vi "List Attribute Names.vi"(7 "Tree ID":string, 8 "Error In":errorcluster, 11 "Tree Manager":refnum<data-value>) -> (0 "Error Out":errorcluster, 1 "Attribute Names":string[](array[string]), 3 "Tree Manager":refnum<data-value>)   [LabVIEW 2017, in "Tree API.lvlib" / "Tree.lvclass"]
doc: "List the attributes names for the specified Tree.\n\nThe list order is preserved as defined."
uses:
  Tree.lvclass
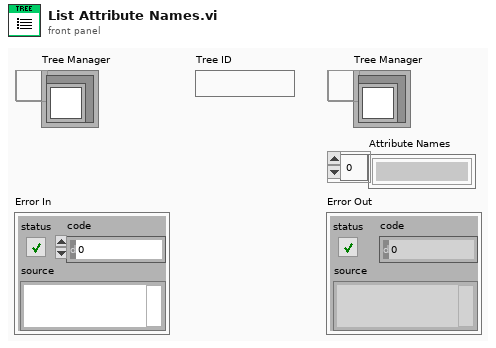
[diagram p1: front panel]
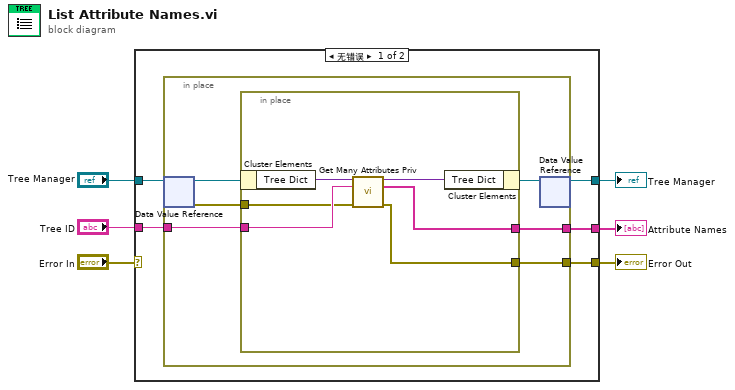
[diagram p0: block diagram]
diagram:
  n1 = case shown="无错误" "Error In" {
    selector: "Error In" -> [_ w24]
    tunnel: "Tree Manager" -> [w11 w25]
    tunnel: [w10 w25] -> w5
    tunnel: [w9 w24] -> w3
    tunnel: "Tree ID" -> [w8 _]
    tunnel: [w7 _] -> w1
    frame No Error {
      n2 = in-place {
        in-place-border: [w16] -> w9
        in-place-border: w8 -> [w13]
        in-place-border: [w12] -> w7
        n3 = in-place-dvr #1(w11) -> (w17:refnum<class "Tree.lvclass">, w14:errorcluster)
        n4 = in-place {
          in-place-border: [w19] -> w16
          in-place-border: w14 -> [w21]
          in-place-border: w13 -> [w22]
          in-place-border: [w18] -> w12
          n5 = in-place-cluster #2(w17) -> ("Tree Dict"=w23:variant)
          n6 = call "Get Many Attributes Priv.vi"("Tree Dictionary In"=w23, "Unique ID"=w22, "error in"=w21) -> ("Tree Dictionary Out"=w20:variant, "Attribute Names"=w18:string[], "error out"=w19:errorcluster)  [unwired: 7 in, 3 out]
          n7 = in-place-cluster #2("Tree Dict"=w20) -> (w15:refnum<class "Tree.lvclass">)
        }
        n8 = in-place-dvr #1(w15) -> (w10:refnum<data-value>)  [unwired: 1 out]
      }
    }
    frame Error {
    }
  }
  "Tree Manager" <- w5
  "Error Out" <- w3
  "Attribute Names" <- w1
